vi "Coerce Port Power Core.vi"(0 "Cal Standard Base in":refnum<class "Cal Standard Base.lvclass">, 5 "Product Name":string, 7 "Port Power":dbl, 9 "Max Allowed Power":dbl=15.0 format="%#_13g", 11 "error in (no error)":errorcluster) -> (4 "Cal Standard Base out":refnum<class "Cal Standard Base.lvclass">, 6 "Coerced Port Power":dbl, 15 "error out":errorcluster)   [LabVIEW 2023, in "RFFixtureCharact.Instruments.lvlib" / "Cal Standard Base.lvclass"]
uses:
  Cal Standard Base.lvclass
  Common/RFCalAndFixtureCharact.Common.lvlib
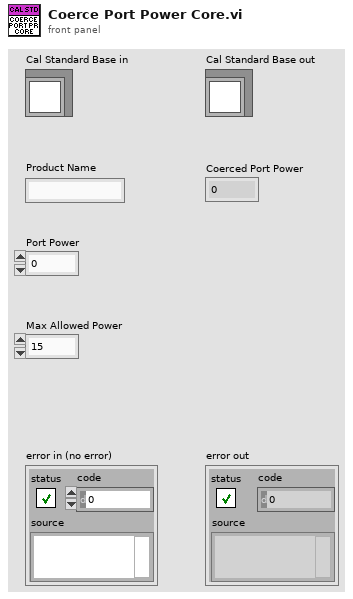
[diagram p1: front panel]
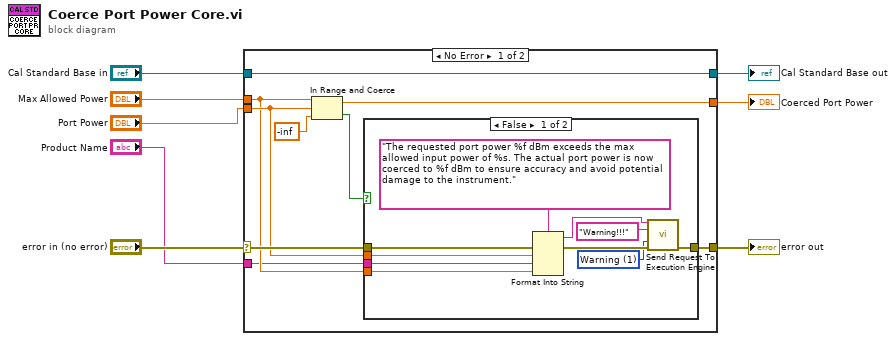
[diagram p0: block diagram]
diagram:
  n1 = case shown="No Error" "error in (no error)" {
    selector: "error in (no error)" -> [w13 w31]
    tunnel: [w14 w31] -> w7
    tunnel: [w17 w30] -> w8
    tunnel: "Cal Standard Base in" -> [w17 w30]
    tunnel: [w16 w29] -> w2
    tunnel: "Port Power" -> [w12 w29]
    tunnel: "Max Allowed Power" -> [w10 _]
    tunnel: "Product Name" -> [w9 _]
    frame No Error {
      n2 = In Range and Coerce(upper limit=w10, x=w12, lower limit=-inf) -> (coerced(x)=w16:dbl, In Range?=w11:bool)
      n3 = case shown="False" w11 {
        tunnel: [w27 w28] -> w14
        tunnel: w13 -> [w25 w28]
        tunnel: w12 -> [w21 _]
        tunnel: w10 -> [w19 _]
        tunnel: w9 -> [w18 _]
        frame False {
          w20 = 1 items=["Info", "Warning", "Error", "Action"] ("RequestContentType")
          n4 = Format Into String(format string="The requested port power %f dBm exceeds the max allowed input power of %s. The actual port power is now coerced to %f dBm to ensure accuracy and avoid potential damage to the instrument.", error in=w25, w21, w18, w19) -> (resulting string=w23:string, error out=w24:errorcluster)  [unwired: 1 in]
          n5 = call "Send Request To Execution Engine.vi"("Request Message"=w23, "Request Header"="Warning!!!", "Request Content Type"=w20, "error in (no error)"=w24) -> ("error out"=w27:errorcluster)  [unwired: 10 in, 1 out]
        }
        frame True {
        }
      }
    }
    frame Error {
    }
  }
  "Cal Standard Base out" <- w8
  "error out" <- w7
  "Coerced Port Power" <- w2
